vi "ConcatenatingArrays.vi"() -> ()   [LabVIEW 2014]
panel:
  out "appended array 2":i32[][](array[numeric])
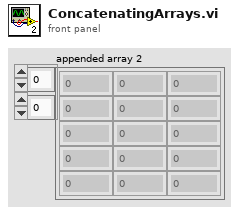
[diagram p1: front panel]
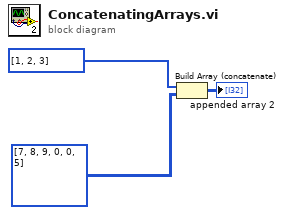
[diagram p0: block diagram]
diagram:
  n1 = Build Array (concatenate)(i32[] [1, 2, 3], i32[][] [[7, 8, 9], [0, 0, 5]]) -> (→"appended array 2":i32[][])
